vi "mouse_ctrl get_mouse_event.vi"(8 "error in (no error)":errorcluster, 11 "mouse_ctrl in":refnum<class "mouse_ctrl.lvclass">) -> (0 "error out":errorcluster, 2 "mouse event":T1, 3 "mouse_ctrl out":refnum<class "mouse_ctrl.lvclass">)   [LabVIEW 2018, in "mouse_ctrl.lvclass"]
uses:
  mouse_ctrl.lvclass
  subVI/mouse_state.ctl
  mouse_ctrl.lvclass/mouse_ctrl.ctl
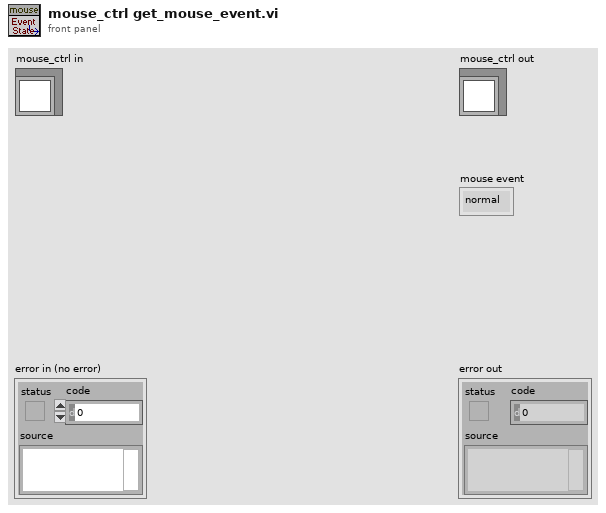
[diagram p1: front panel]
types:
  T1 = typedef "mouse_state.ctl" = enum16{"normal", "mouse down", "calc"}
  T2 = typedef "mouse_ctrl.lvclass/mouse_state.ctl" = enum16{"normal", "mouse down", "calc"}
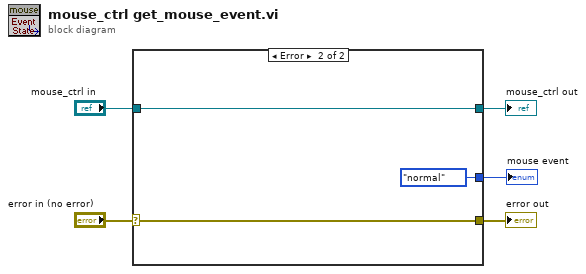
[diagram p0: block diagram]
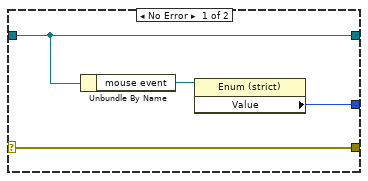
[diagram p2: hidden frame]
diagram:
  n1 = case shown="Error" "error in (no error)" {
    selector: "error in (no error)" -> [w9 w12]
    tunnel: [w9 w12] -> w4
    tunnel: [w8 w11] -> w2
    tunnel: "mouse_ctrl in" -> [w8 w11]
    tunnel: [w6 mouse_state."normal" ("Value")] -> w1
    frame No Error {
      n2 = Unbundle By Name(w8) -> ("mouse event"=w7:refnum<vi>)
      n3 = property class="Enum (strict)"(reference=w7) -> ("Value"=w6:T2)  [unwired: 1 in, 2 out]
    }
    frame Error {
    }
  }
  "error out" <- w4
  "mouse_ctrl out" <- w2
  "mouse event" <- w1
